vi "DAC Save Results.vi"(8 "error in":errorcluster, 9 "Log Details?":bool, 10 "tdms file":refnum<k34>, 11 "DAC Vacum Pressure in":refnum<class "DAC Vacum Pressure.lvclass">) -> (0 "error out":errorcluster)   [LabVIEW 2019, in "DAC.lvlib" / "DAC Vacum Pressure.lvclass"]
uses:
  DAC Vacum Pressure.lvclass
  C:/Users/krio/Documents/LV_Projects/test-stand/App/DAC/DAC.lvclass
  DAC.lvclass/DAC.ctl
  DAC Vacum Pressure.lvclass/DAC Vacum Pressure.ctl
  DAC.lvclass
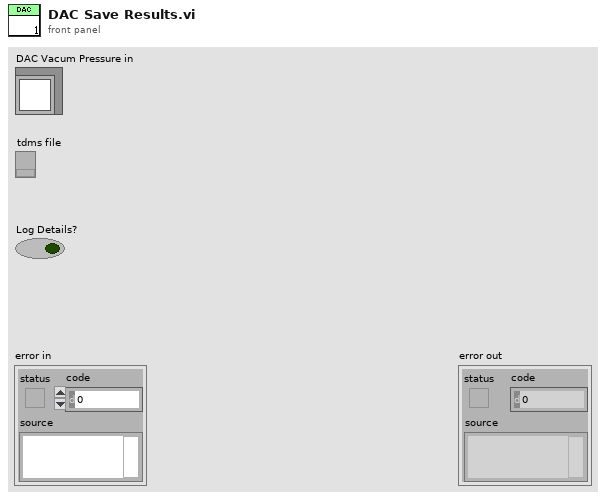
[diagram p1: front panel]
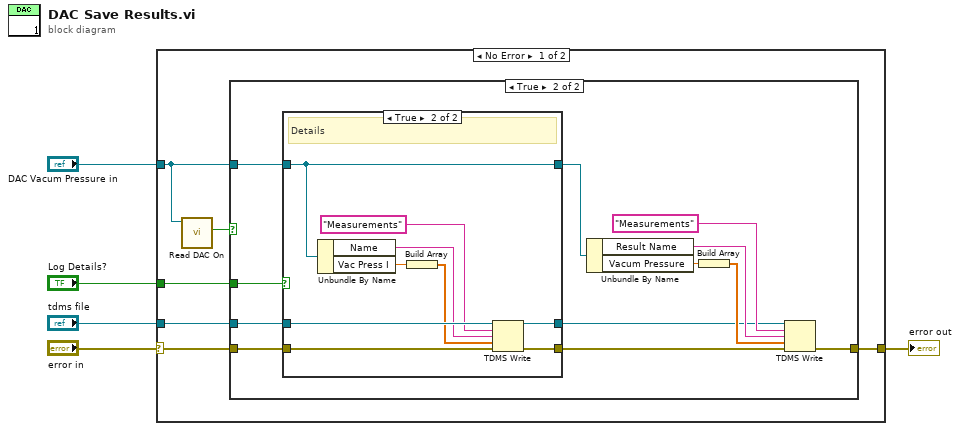
[diagram p0: block diagram]
diagram:
  n1 = case shown="No Error" "error in" {
    selector: "error in" -> [w8 w37]
    tunnel: "DAC Vacum Pressure in" -> [w11 _]
    tunnel: "tdms file" -> [w9 _]
    tunnel: [w7 w37] -> w3
    tunnel: "Log Details?" -> [w6 _]
    frame No Error {
      n2 = call "Read DAC On.vi"("DAC in"=w11) -> ("DAC On"=w10:bool)  [unwired: 8 in, 2 out]
      n3 = case shown="True" w10 {
        tunnel: w11 -> [_ w17]
        tunnel: w9 -> [_ w15]
        tunnel: w8 -> [w12 w16]
        tunnel: [w12 w13] -> w7
        tunnel: w6 -> [_ w14]
        frame False {
        }
        frame True {
          n4 = case shown="True" w14 {
            tunnel: w15 -> [w26 w36]
            tunnel: w16 -> [w27 w31]
            tunnel: w17 -> [w25 w28]
            tunnel: [w27 w30] -> w19
            tunnel: [w26 w29] -> w20
            tunnel: [w25 w28] -> w18
            frame False {
            }
            frame True {
              # "Details"
              n5 = Unbundle By Name(w28) -> ("Name"=w33:string, "Vac Press I"=w35:dbl)
              n6 = Build Array(w35) -> (w34:dbl[])
              n7 = TDMS Write(0:w36, 5:"Measurements" ("group name in (Untitled)"), 7:w33, 9:w34, 11:w31) -> (4:w29:refnum<k34>, 15:w30:errorcluster)  [unwired: 1 in, 2 out]
            }
          }
          n8 = Unbundle By Name(w18) -> ("Result Name"=w22:string, "Vacum Pressure"=w24:dbl)
          n9 = Build Array(w24) -> (w23:dbl[])
          n10 = TDMS Write(0:w20, 5:"Measurements" ("group name in (Untitled)"), 7:w22, 9:w23, 11:w19) -> (15:w13:errorcluster)  [unwired: 1 in, 3 out]
        }
      }
    }
    frame Error {
    }
  }
  "error out" <- w3
